vi "Display Message Dialog.vi"(8 "error in":errorcluster, 11 "Message to display":string) -> (0 "error out":errorcluster)   [LabVIEW 2019, in "SEECD System Explorer.lvlib"]
uses:
  SEECD System Explorer.lvlib
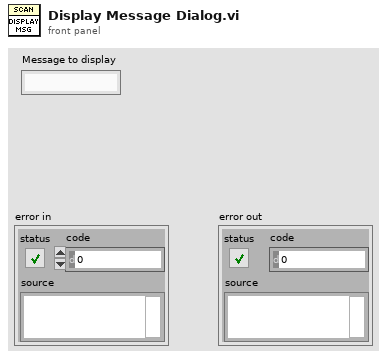
[diagram p1: front panel]
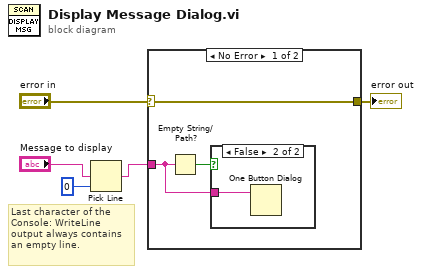
[diagram p0: block diagram]
diagram:
  # "Last character of the\nConsole: WriteLine\noutput always contains\nan empty line."
  n1 = Pick Line(multi-line string="Message to display", line index=0) -> (output string=w2:string)  [unwired: 1 in]
  n2 = case shown="No Error" "error in" {
    selector: "error in" -> [w8 w10]
    tunnel: [w8 w10] -> w4
    tunnel: w2 -> [w6 _]
    frame No Error {
      n3 = Empty String/Path?(string/path=w6) -> (empty?=w7:bool)
      n4 = case shown="False" w7 {
        tunnel: w6 -> [_ w9]
        frame True {
        }
        frame False {
          n5 = One Button Dialog(message=w9) -> ()  [unwired: 1 in, 1 out]
        }
      }
    }
    frame Error {
    }
  }
  "error out" <- w4
